vi "Elapsed Time.vi"(9 "error in (no error)":errorcluster, 10 "Delay Time (s)":dbl=3.0) -> ()   [LabVIEW 2015]
panel:
  out "Relative Time":u32
  in  "Boolean":bool
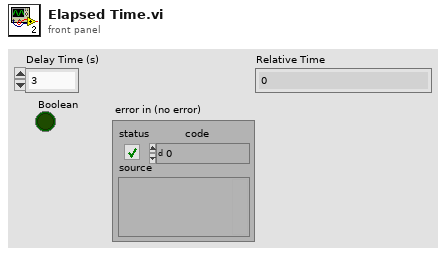
[diagram p1: front panel]
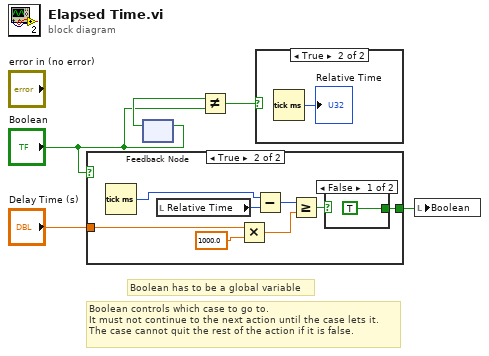
[diagram p0: block diagram]
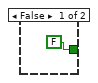
[diagram p3: hidden frame]
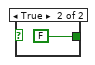
[diagram p4: hidden frame]
diagram:
  # "Boolean controls which case to go to. \nIt must not continue to the next action until the case lets it.\nThe case cannot quit the rest of the action if it is false."
  # "Boolean has to be a global variable"
  n1 = case shown="True" "Boolean" {
    tunnel: "Delay Time (s)" -> [_ w9]
    tunnel: [FALSE w12] -> w4
    frame False {
    }
    frame True {
      n2 = Tick Count (ms)() -> (millisecond timer value=w7:u32)
      n3 = local read "Relative Time"() -> (w11:u32)
      n4 = Multiply(x=w9, y=1000.0) -> (x*y=w10:dbl)
      n5 = Subtract(x=w7, y=w11) -> (x-y=w14:u32)
      n6 = Greater Or Equal?(x=w14, y=w10) -> (x >= y?=w13:bool)
      n7 = case shown="False" w13 {
        tunnel: [TRUE FALSE] -> w12
        frame False {
        }
        frame True {
        }
      }
    }
  }
  n8 = feedback-in #1("Boolean") -> ()
  n9 = feedback #1() -> (w3:bool)  [unwired: 1 in]
  n10 = Not Equal?(x=w3, y="Boolean") -> (x != y?=w1:bool)
  n11 = case shown="True" w1 {
    frame False {
    }
    frame True {
      n12 = Tick Count (ms)() -> (millisecond timer value=→"Relative Time":u32)
    }
  }
  n13 = local write "Boolean"(w4) -> ()
